vi "HandleDigitalInputModuleNames.vi"(8 "Error In":errorcluster, 10 "Port Name In":string, 11 "Data In":string) -> (0 "Error Out":errorcluster, 1 "Meas Name":string, 2 "Module and CH":string, 3 "Channel":string)   [LabVIEW 2011]
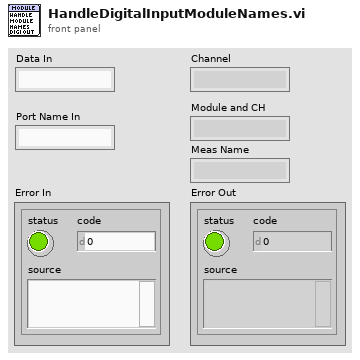
[diagram p1: front panel]
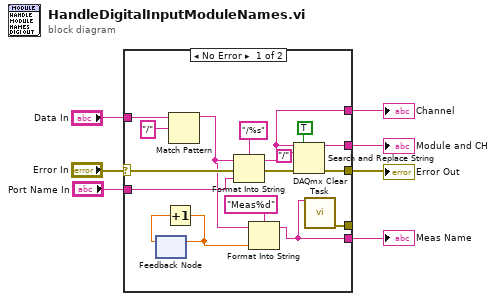
[diagram p0: block diagram]
diagram:
  n1 = case shown="No Error" "Error In" {
    selector: "Error In" -> [w15 w25]
    tunnel: [w11 _] -> w5
    tunnel: [w24 _] -> w6
    tunnel: "Data In" -> [w21 _]
    tunnel: "Port Name In" -> [w20 _]
    tunnel: [w16 w25] -> w4
    tunnel: [w10 _] -> w7
    tunnel: [w9 _] -> _
    frame No Error {
      n2 = feedback #1() -> (w14:dbl)  [unwired: 1 in]
      n3 = Increment(x=w14) -> (x+1=w13:dbl)
      n4 = feedback-in #1(w13) -> ()
      n5 = Match Pattern(string=w21, regular expression="/") -> (before substring=w8:string)  [unwired: 1 in, 3 out]
      n6 = Format Into String(format string="/%s", initial string=w8, error in=w15, w20) -> (resulting string=w24:string, error out=w17:errorcluster)
      n7 = Format Into String(format string="Meas%d", initial string=w8, w13) -> (resulting string=w10:string)  [unwired: 1 in, 1 out]
      n8 = Search and Replace String(replace all?=TRUE ("replace all? (F)"), input string=w24, search string="/", error in=w17) -> (result string=w11:string, error out=w16:errorcluster)  [unwired: 4 in, 2 out]
      n9 = call <vilib>:"DAQmx Clear Task.vi"("task in"=w10) -> ("error out"=w9:errorcluster)  [unwired: 14 in]
    }
    frame Error {
    }
  }
  "Module and CH" <- w5
  "Channel" <- w6
  "Error Out" <- w4
  "Meas Name" <- w7
